vi "FindMostRecentCalFile.vi"(0 "DIR_IN":path=path "C:/RageATE/Automated Tests/Tetra WAM/PRODUCTION/Test Benches/WAM_PROD_TEST-1/Calibration Files", 11 "error in (no error)":errorcluster, 12 "Test Bench (for filename match)":string(combo)="WAM_PROD_TEST-2", 13 "line index":i32(ring) items=["INPUT", "OUTPUT"], 14 "IsRuntime?":bool) -> (3 "Success?(t)":bool, 4 "cal_path_out":path, 15 "error out":errorcluster)   [LabVIEW 2018]
uses:
  406562c1-697f-4648-b42d-40e5e1d0334e.vi
  <vilib>/Array/Sort 2D Array - Pop Stack.vi
  <vilib>/Array/Sort 2D Array - Push Stack.vi
panel:
  out "Array 2":string[](array[string])
  out "Newest File":string
  out "sorted 2D array":string[][](array[string])
  out "Array":string[](array[string])
  out "Time(num)":dbl[](array[numeric])
  out "Timestamp":timestamp[](array[timestamp])
  out "Filtered Files":string[](array[string])
  out "array":string[](array[string])
  out "standard output":string
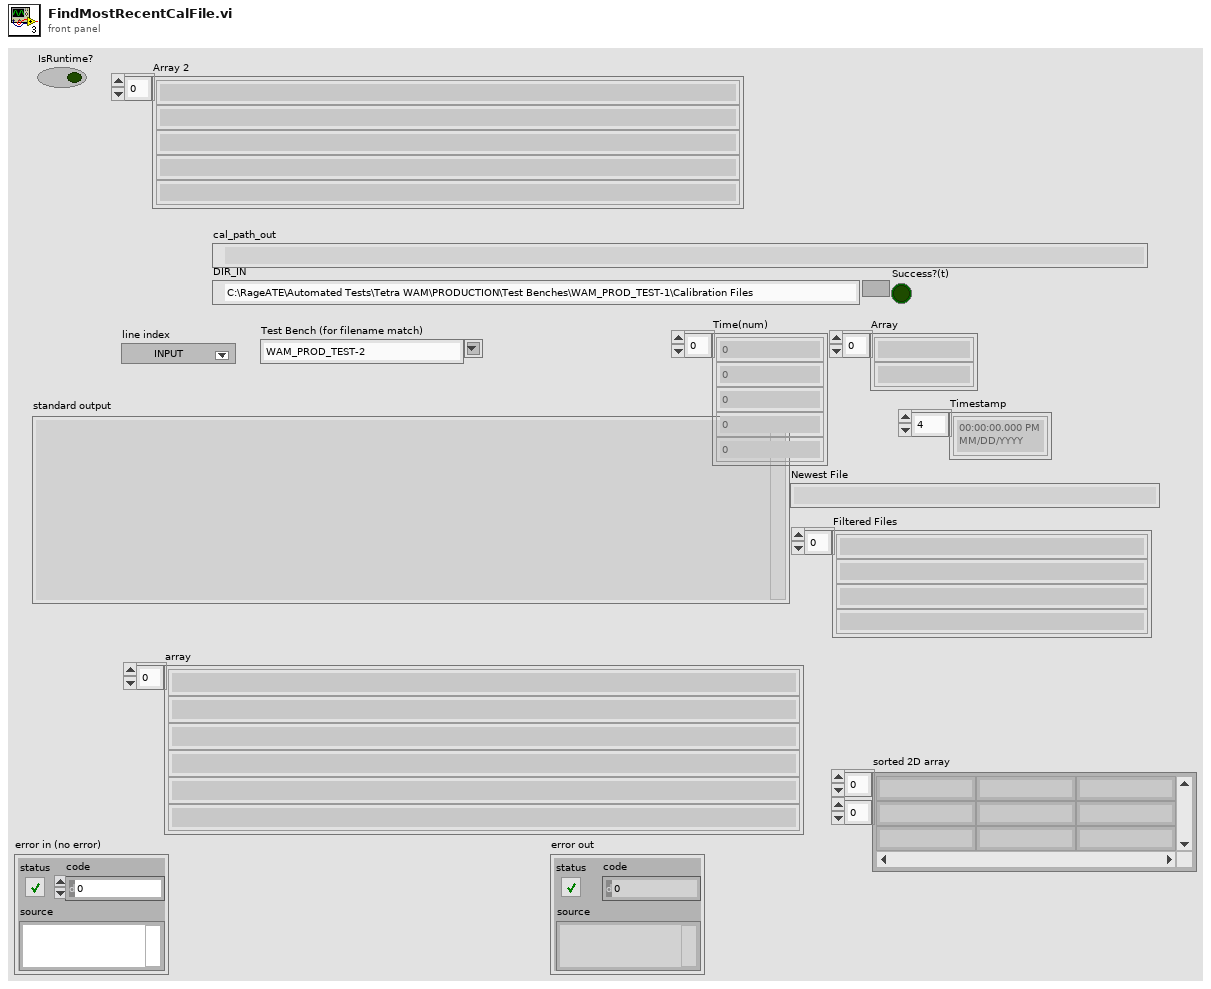
[diagram p1: front panel]
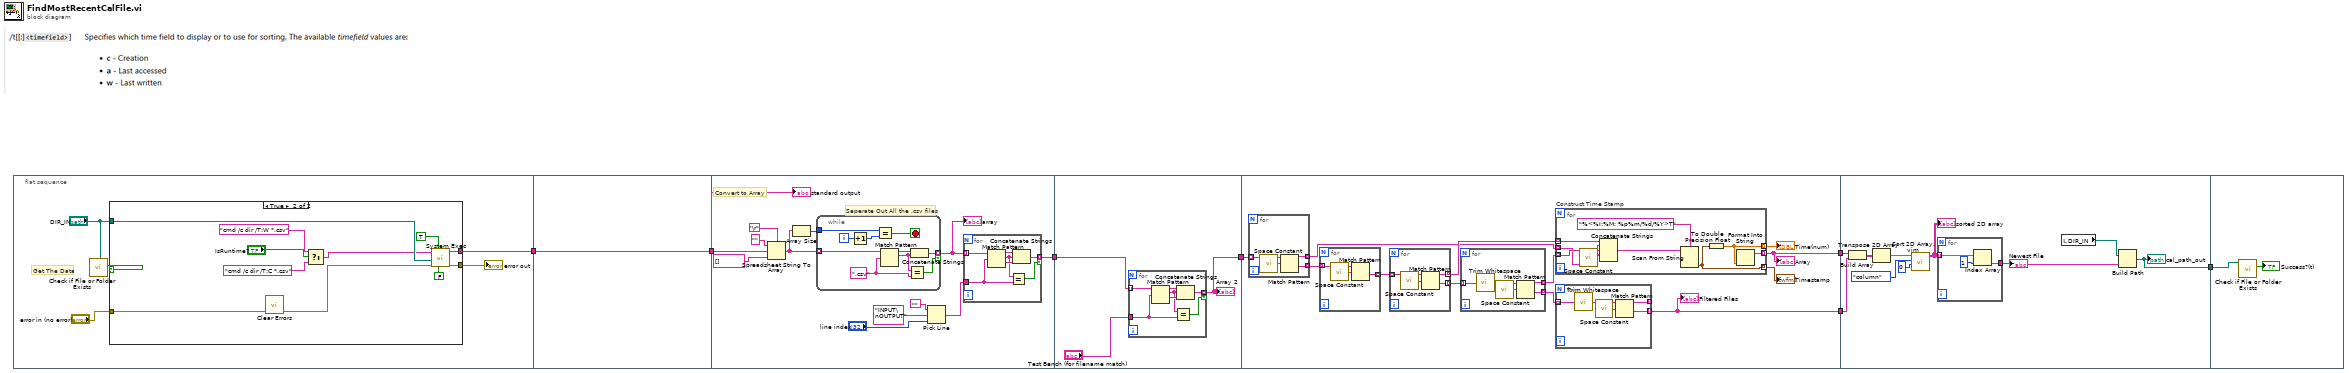
[diagram p0: block diagram]
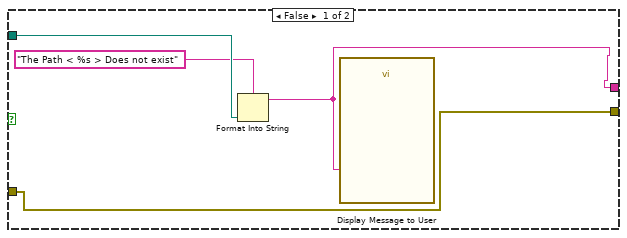
[diagram p2: hidden frame]
diagram:
  n1 = flat-sequence {
    tunnel: [w12] -> w4
    tunnel: w4 -> [w28]
    tunnel: [w28] -> w3
    tunnel: w3 -> [w38]
    tunnel: [w33] -> w2
    tunnel: w2 -> [w60]
    tunnel: [w58] -> w1
    tunnel: w1 -> [w79]
    tunnel: [w70] -> w7
    tunnel: [w68] -> w6
    tunnel: w7 -> [w118]
    tunnel: w6 -> [w119]
    tunnel: [w110] -> w5
    tunnel: w5 -> [w124]
    frame #0 {
      # "Get The Data"
      n2 = call <vilib>:"Check if File or Folder Exists.vi"("path"="DIR_IN") -> ("file or folder exists?"=w9:bool)  [unwired: 8 in, 2 out]
      n3 = case shown="True" w9 {
        tunnel: [w13 w25] -> w12
        tunnel: [w15 w23] -> w11
        tunnel: "DIR_IN" -> [w16 w22]
        tunnel: "error in (no error)" -> [w15 w21]
        frame False {
          n4 = Format Into String(format string="The Path < %s > Does not exist", w16) -> (resulting string=w13:string)  [unwired: 2 in, 1 out]
          n5 = call "Display Message to User"("Message"=w13) -> ()  [unwired: 9 in, 2 out]
        }
        frame True {
          n6 = call <vilib>:"Clear Errors.vi"("error in (no error)"=w21) -> ("error out"=w24:errorcluster)  [unwired: 5 in, 1 out]
          n7 = Select(t="cmd /c dir /T:W *.csv" ("command line"), s="IsRuntime?", f="cmd /c dir /T:C *.csv" ("command line")) -> (s? t:f=w19:string)
          n8 = call <vilib>:"System Exec.vi"("run minimized? (F)"=FALSE, "wait until completion? (T)"=TRUE, "error in (no error)"=w24, "working directory"=w22, "command line"=w19) -> ("error out"=w23:errorcluster, "standard output"=w25:string)  [unwired: 3 in, 2 out]
        }
      }
      "error out" <- w11
    }
    frame #1 {
    }
    frame #2 {
      # "Convert to Array"
      # "Seperate Out All the .csv files"
      n9 = Spreadsheet String To Array(delimiter (Tab)="\r", format string="", spreadsheet string=w38, array type (2D Dbl)=string[] []) -> (array=w36:string[])
      n10 = Array Size(array=w36) -> (size(s)=w35:i32)
      n11 = while {
        tunnel: w36 -> [w57] mode=indexing
        tunnel: [w55] -> w34 mode=indexing if=w54
        tunnel: w35 -> [w50]
        i -> [w49]
        stop <- w51 stop-if-true
        w52 = ".csv" ("regular expression")
        n12 = Increment(x=w49) -> (x+1=w48:i32)
        n13 = Equal?(x=w50, y=w48) -> (x = y?=w51:bool)
        n14 = Match Pattern(string=w57, regular expression=w52) -> (before substring=w56:string, match substring=w53:string)  [unwired: 1 in, 2 out]
        n15 = Equal?(x=w53, y=w52) -> (x = y?=w54:bool)
        n16 = Concatenate Strings(w56, w53) -> (w55:string)
      }
      "array" <- w34
      n17 = Pick Line(string ("")="", multi-line string="INPUT\nOUTPUT", line index="line index") -> (output string=w30:string)
      n18 = for {
        tunnel: w34 -> [w47] mode=indexing
        tunnel: w30 -> [w43]
        tunnel: [w42] -> w33 mode=indexing if=w41
        n19 = Match Pattern(string=w47, regular expression=w43) -> (before substring=w46:string, match substring=w44:string, after substring=w45:string)  [unwired: 1 in, 1 out]
        n20 = Equal?(x=w44, y=w43) -> (x = y?=w41:bool)
        n21 = Concatenate Strings(w46, w44, w45) -> (w42:string)
      }
      "standard output" <- w38
    }
    frame #3 {
      n22 = for {
        tunnel: w60 -> [w67] mode=indexing
        tunnel: "Test Bench (for filename match)" -> [w63]
        tunnel: [w62] -> w58 mode=indexing if=w61
        n23 = Match Pattern(string=w67, regular expression=w63) -> (before substring=w66:string, match substring=w64:string, after substring=w65:string)  [unwired: 1 in, 1 out]
        n24 = Equal?(x=w64, y=w63) -> (x = y?=w61:bool)
        n25 = Concatenate Strings(w66, w64, w65) -> (w62:string)
      }
      "Array 2" <- w58
    }
    frame #4 {
      n26 = for {
        tunnel: w79 -> [w109] mode=indexing
        tunnel: [w107] -> w73 mode=indexing
        tunnel: [w106] -> w78 mode=indexing
        n27 = call <vilib>:"Space Constant.vi"() -> ("String"=w108:string)
        n28 = Match Pattern(string=w109, regular expression=w108) -> (before substring=w107:string, after substring=w106:string)  [unwired: 1 in, 2 out]
      }
      n29 = for {
        tunnel: w78 -> [w105] mode=indexing
        tunnel: [w103] -> w77 mode=indexing
        n30 = call <vilib>:"Space Constant.vi"() -> ("String"=w104:string)
        n31 = Match Pattern(string=w105, regular expression=w104) -> (after substring=w103:string)  [unwired: 1 in, 3 out]
      }
      n32 = for {
        tunnel: w77 -> [w102] mode=indexing
        tunnel: [w100] -> w74 mode=indexing
        tunnel: [w99] -> w76 mode=indexing
        n33 = call <vilib>:"Space Constant.vi"() -> ("String"=w101:string)
        n34 = Match Pattern(string=w102, regular expression=w101) -> (before substring=w100:string, after substring=w99:string)  [unwired: 1 in, 2 out]
      }
      n35 = for {
        tunnel: w76 -> [w98] mode=indexing
        tunnel: [w96] -> w72 mode=indexing
        tunnel: [w95] -> w75 mode=indexing
        n36 = call <vilib>:"Trim Whitespace.vi"("string"=w98) -> ("trimmed string"=w94:string)  [unwired: 1 in]
        n37 = call <vilib>:"Space Constant.vi"() -> ("String"=w97:string)
        n38 = Match Pattern(string=w94, regular expression=w97) -> (before substring=w96:string, after substring=w95:string)  [unwired: 1 in, 2 out]
      }
      n39 = for "Construct Time Stamp" {
        tunnel: w74 -> [w86] mode=indexing
        tunnel: w73 -> [w83] mode=indexing
        tunnel: [w82] -> w71 mode=indexing
        tunnel: w72 -> [w85] mode=indexing
        tunnel: [w81] -> w69 mode=indexing
        tunnel: [w80] -> w68 mode=indexing
        n40 = call <vilib>:"Space Constant.vi"() -> ("String"=w84:string)
        n41 = Concatenate Strings(w86, w84, w85, w84, w83) -> (w88:string)
        n42 = Scan From String(format string="%<%I:%M: %p%m/%d/%Y>T", input string=w88) -> (output 1=w82:timestamp)  [unwired: 3 in, 3 out]
        n43 = To Double Precision Float(number=w82) -> (double precision float=w81:dbl)
        n44 = Format Into String(w81) -> (resulting string=w80:string)  [unwired: 3 in, 1 out]
      }
      "Timestamp" <- w71
      "Time(num)" <- w69
      "Array" <- w68
      n45 = for {
        tunnel: w75 -> [w93] mode=indexing
        tunnel: [w91] -> _ mode=indexing
        tunnel: [w90] -> w70 mode=indexing
        n46 = call <vilib>:"Trim Whitespace.vi"("string"=w93) -> ("trimmed string"=w89:string)  [unwired: 1 in]
        n47 = call <vilib>:"Space Constant.vi"() -> ("String"=w92:string)
        n48 = Match Pattern(string=w89, regular expression=w92) -> (before substring=w91:string, after substring=w90:string)  [unwired: 1 in, 2 out]
      }
      "Filtered Files" <- w70
    }
    frame #5 {
      n49 = Build Array(w119, w118) -> (w117:string[][])
      n50 = Transpose 2D Array(2D array=w117) -> (transposed array=w116:string[][])
      n51 = call "Sort 2D Array.vim"("index"=0, "dimension to index (column)"=enum16{"column", "row"}."column", "2D array"=w116) -> ("sorted 2D array"=w113:string[][])  [unwired: 7 in, 1 out]
      "sorted 2D array" <- w113
      n52 = for {
        tunnel: w113 -> [w122] mode=indexing
        tunnel: [w120] -> w111
        n53 = Index Array(array=w122, index=1) -> (element=w120:string)
      }
      "Newest File" <- w111
      n54 = local read "DIR_IN"() -> (w112:path)
      n55 = Build Path(base path=w112, name or relative path=w111) -> (appended path=w110:path)
      "cal_path_out" <- w110
    }
    frame #6 {
      n56 = call <vilib>:"Check if File or Folder Exists.vi"("path"=w124) -> ("file or folder exists?"=→"Success?(t)":bool)  [unwired: 8 in, 2 out]
    }
  }
